vi "Write title.vi"(8 "error in (no error)":errorcluster, 10 "title":string, 11 "[V] Waveform in":refnum<class "[V] Waveform.lvclass">) -> (0 "error out":errorcluster, 3 "[V] Waveform out":refnum<class "[V] Waveform.lvclass">)   [LabVIEW 2023, in "[V] Waveform.lvlib" / "[V] Waveform.lvclass"]
uses:
  [V] Waveform.lvclass
  [V] Waveform.lvclass/[V] Waveform.ctl
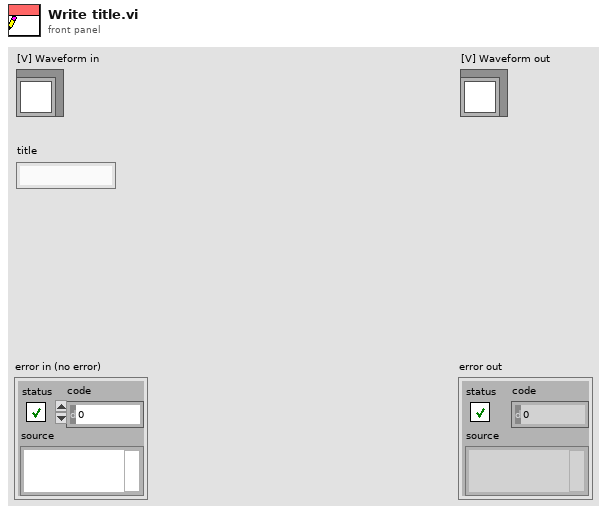
[diagram p1: front panel]
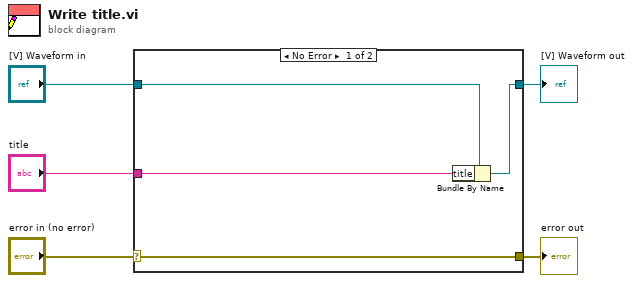
[diagram p0: block diagram]
diagram:
  n1 = case shown="No Error" "error in (no error)" {
    selector: "error in (no error)" -> [w9 w10]
    tunnel: [w9 w10] -> w4
    tunnel: [w7 w11] -> w2
    tunnel: "[V] Waveform in" -> [w8 w11]
    tunnel: "title" -> [w6 _]
    frame No Error {
      n2 = Bundle By Name(cluster=w8, "title"=w6) -> (w7:refnum<class "[V] Waveform.lvclass">)
    }
    frame Error {
    }
  }
  "error out" <- w4
  "[V] Waveform out" <- w2
